vi "Set Property.vi"(8 "error in (no error)":errorcluster, 9 "Value":dbl, 10 "Property":string, 11 "Channel in":refnum<class "Channel.lvclass">) -> (0 "error out":errorcluster, 3 "Channel out":refnum<class "Channel.lvclass">)   [LabVIEW 2015, in "Channel.lvclass"]
uses:
  Channel.lvclass
  Channel.lvclass/Channel.ctl
  Level/Level.lvclass/Level.ctl
  Level/Write Level.vi
  <vilib>/regexp/Match Regular Expression.xnode
  Waveforms/Waveform/Waveform.lvclass
  Modulations/AM/AM.lvclass
  Gate/Gate.lvclass
  Filter/Filter.lvclass
  Level/Level.lvclass
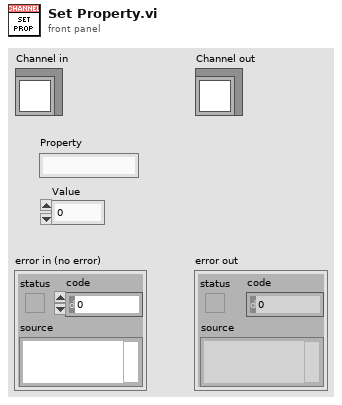
[diagram p1: front panel]
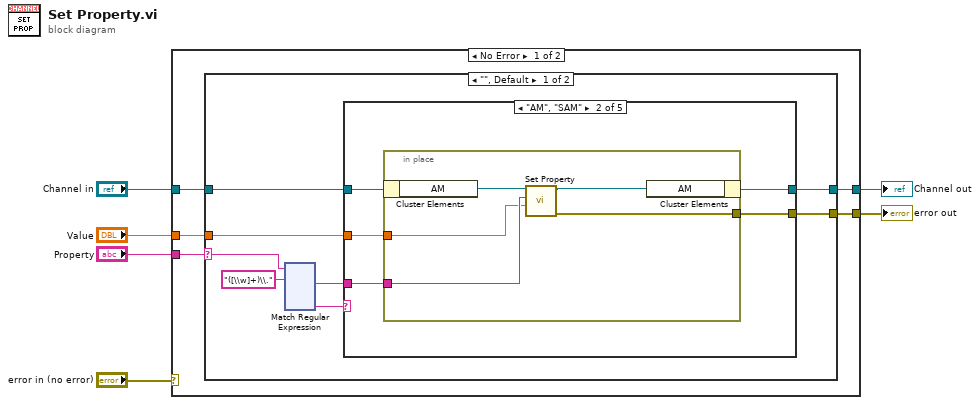
[diagram p0: block diagram]
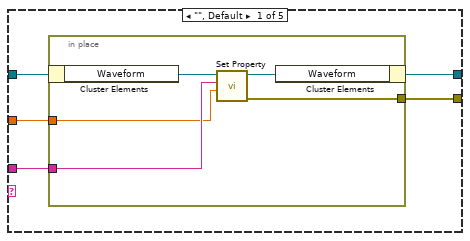
[diagram p2: hidden frame]
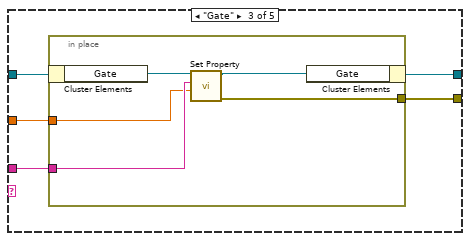
[diagram p3: hidden frame]
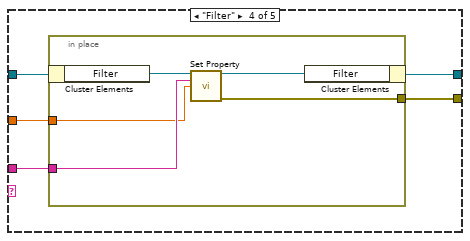
[diagram p4: hidden frame]
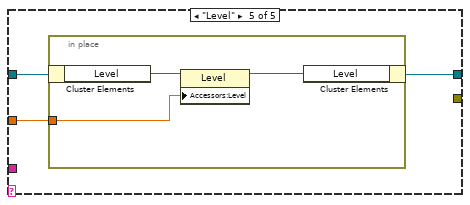
[diagram p5: hidden frame]
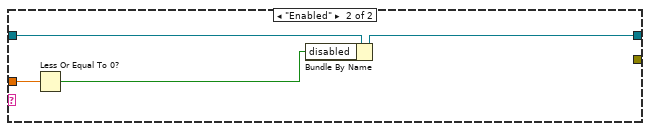
[diagram p6: hidden frame]
diagram:
  n1 = case shown="No Error" "error in (no error)" {
    selector: "error in (no error)" -> [_ w187]
    tunnel: [w8 w187] -> w5
    tunnel: [w9 w186] -> w3
    tunnel: "Channel in" -> [w10 w186]
    tunnel: "Property" -> [w7 _]
    tunnel: "Value" -> [w11 _]
    frame No Error {
      n2 = case shown="\"\", Default" w7 {
        selector: w7 -> [w12 _]
        tunnel: w11 -> [w19 w183]
        tunnel: w10 -> [w15 w185]
        tunnel: [w14 w184] -> w9
        tunnel: [w13 _] -> w8
        frame "", Default {
          n3 = xnode "Match Regular Expression"("input string"=w12, "regular expression"="([\\w]+)\\.") -> ("after match"=w16:string, "submatch 1"=w17:string)  [unwired: 4 in, 4 out]
          n4 = case shown="\"AM\", \"SAM\"" w17 {
            tunnel: [w22 w32 w42 w52 w60] -> w14
            tunnel: w19 -> [w24 w34 w44 w54 w62]
            tunnel: w16 -> [w21 w31 w41 w51 _]
            tunnel: w15 -> [w23 w33 w43 w53 w61]
            tunnel: [w20 w30 w40 w50 _] -> w13
            frame "", Default {
              n5 = in-place {
                in-place-border: w24 -> [w26]
                in-place-border: w21 -> [w27]
                in-place-border: [w25] -> w20
                n6 = in-place-cluster #1(w23) -> ("Waveform"=w29:refnum<class "Waveform.lvclass">)
                n7 = call-dynamic "Set Property.vi"("Value"=w26, "Property"=w27, "Waveform in"=w29) -> ("error out"=w25:errorcluster, "Waveform out"=w28:refnum<class "Waveform.lvclass">)  [unwired: 7 in]
                n8 = in-place-cluster #1("Waveform"=w28) -> (w22:refnum<class "Channel.lvclass">)
              }
            }
            frame "AM", "SAM" {
              n9 = in-place {
                in-place-border: w34 -> [w37]
                in-place-border: w31 -> [w38]
                in-place-border: [w35] -> w30
                n10 = in-place-cluster #2(w33) -> ("AM"=w39:refnum<class "AM.lvclass">)
                n11 = call-dynamic "Set Property.vi"("Value"=w37, "Property"=w38, "AM in"=w39) -> ("error out"=w35:errorcluster, "AM out"=w36:refnum<class "AM.lvclass">)  [unwired: 7 in]
                n12 = in-place-cluster #2("AM"=w36) -> (w32:refnum<class "Channel.lvclass">)
              }
            }
            frame "Gate" {
              n13 = in-place {
                in-place-border: w44 -> [w47]
                in-place-border: w41 -> [w48]
                in-place-border: [w45] -> w40
                n14 = in-place-cluster #3(w43) -> ("Gate"=w49:refnum<class "Gate.lvclass">)
                n15 = call "Set Property.vi"("Value"=w47, "Property"=w48, "Gate in"=w49) -> ("error out"=w45:errorcluster, "Gate out"=w46:refnum<class "Gate.lvclass">)  [unwired: 7 in]
                n16 = in-place-cluster #3("Gate"=w46) -> (w42:refnum<class "Channel.lvclass">)
              }
            }
            frame "Filter" {
              n17 = in-place {
                in-place-border: w54 -> [w55]
                in-place-border: w51 -> [w58]
                in-place-border: [w56] -> w50
                n18 = in-place-cluster #4(w53) -> ("Filter"=w59:refnum<class "Filter.lvclass">)
                n19 = call "Set Property.vi"("Filter in"=w59, "Property"=w58, "Value"=w55) -> ("Filter out"=w57:refnum<class "Filter.lvclass">, "error out"=w56:errorcluster)  [unwired: 11 in]
                n20 = in-place-cluster #4("Filter"=w57) -> (w52:refnum<class "Channel.lvclass">)
              }
            }
            frame "Level" {
              n21 = in-place {
                in-place-border: w62 -> [w65]
                n22 = in-place-cluster #5(w61) -> ("Level"=w64:refnum<class "Level.lvclass">)
                n23 = property class="Level"(reference=w64, "Accessors:Level"=w65) -> (reference out=w63:refnum<class "Level.lvclass">)  [unwired: 1 in, 1 out]
                n24 = in-place-cluster #5("Level"=w63) -> (w60:refnum<class "Channel.lvclass">)
              }
            }
          }
        }
        frame "Enabled" {
          n25 = Less Or Equal To 0?(x=w183) -> (x <= 0?=w182:bool)
          n26 = Bundle By Name(cluster=w185, "disabled"=w182) -> (w184:refnum<class "Channel.lvclass">)
        }
      }
    }
    frame Error {
    }
  }
  "error out" <- w5
  "Channel out" <- w3
